vi "Get Resource ID.vi"(4 "PWM in":refnum<class "PWM.lvclass">) -> (7 "Resource ID":string)   [LabVIEW 2024, in "CTI.lvlib" / "PWM.lvclass"]
uses:
  PWM.lvclass
  PWM.lvclass/PWM.ctl
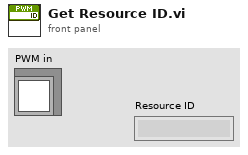
[diagram p1: front panel]
types:
  T1 = typedef "CTI.lvlib/GPIO Number.ctl" = i8
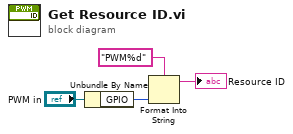
[diagram p0: block diagram]
diagram:
  n1 = Unbundle By Name("PWM in") -> ("GPIO"=w3:T1)
  n2 = Format Into String(format string="PWM%d", w3) -> (resulting string=→"Resource ID":string)  [unwired: 2 in, 1 out]
